vi "Quick Usb Read Setting.vi"(8 "error in (no error)":errorcluster, 9 "value":u16, 10 "address":u16, 11 "hDevice":u32) -> (0 "error out":errorcluster, 1 "value out":u16, 2 "function return":i32, 3 "hDevice out":u32)   [LabVIEW 2011, in "QuickUSB.lvlib"]
doc: "QUSBLIB QRETURN QuickUsbReadSetting(\n QHANDLE hDevice, \n QWORD address, \n PQWORD value\n);"
uses:
  QuickUSB.lvlib
  QuickUSB.dll
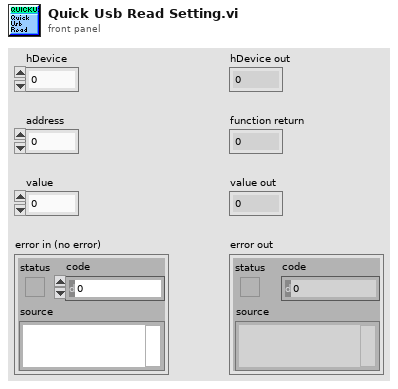
[diagram p1: front panel]
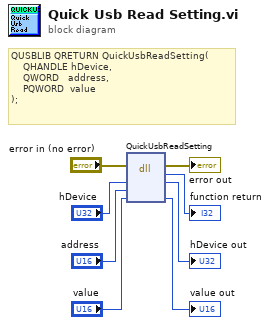
[diagram p0: block diagram]
diagram:
  # "QUSBLIB QRETURN QuickUsbReadSetting(\n    QHANDLE hDevice, \n    QWORD   address, \n    PQWORD  value\n);"
  n1 = dll-call lib="C:/QuickUSB/QuickUSB.*" fn="QuickUsbReadSetting"(error in="error in (no error)", "hDevice"="hDevice", "address"="address", "value"="value") -> (error out=→"error out":errorcluster, →"function return":i32, "hDevice"=→"hDevice out":u32, "value"=→"value out":u16)  [unwired: 3 in, 1 out]
